vi "board_new_board.vi"() -> (0 "chess pieces":variant, 1 "new board":picture[][](array[picture]))   [LabVIEW 2014]
doc: "Generates an 8x8 array of pictures that depicts a chess board with pieces in their starting positions (white on bottom)."
uses:
  board_piece_names.ctl
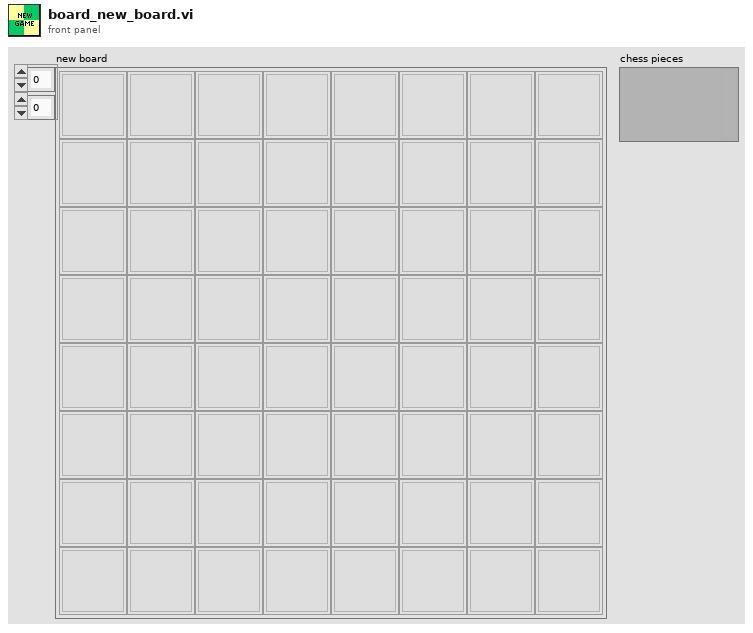
[diagram p1: front panel]
types:
  T1 = typedef "board_piece_names.ctl" = enum16{"Bblk", "Bwht", "Kblk", "Kwht", "Nblk", "Nwht", "Pblk", "Pwht", "Qblk", "Qwht", "Rblk", "Rwht"}
  T2 = typedef "imagedata.ctl" = cluster{"image type":i32, "image depth":i32, "image":u8[], "mask":u8[], "colors":u32[], "Rectangle":cluster{"left":i16, "top":i16, "right":i16, "bottom":i16}}
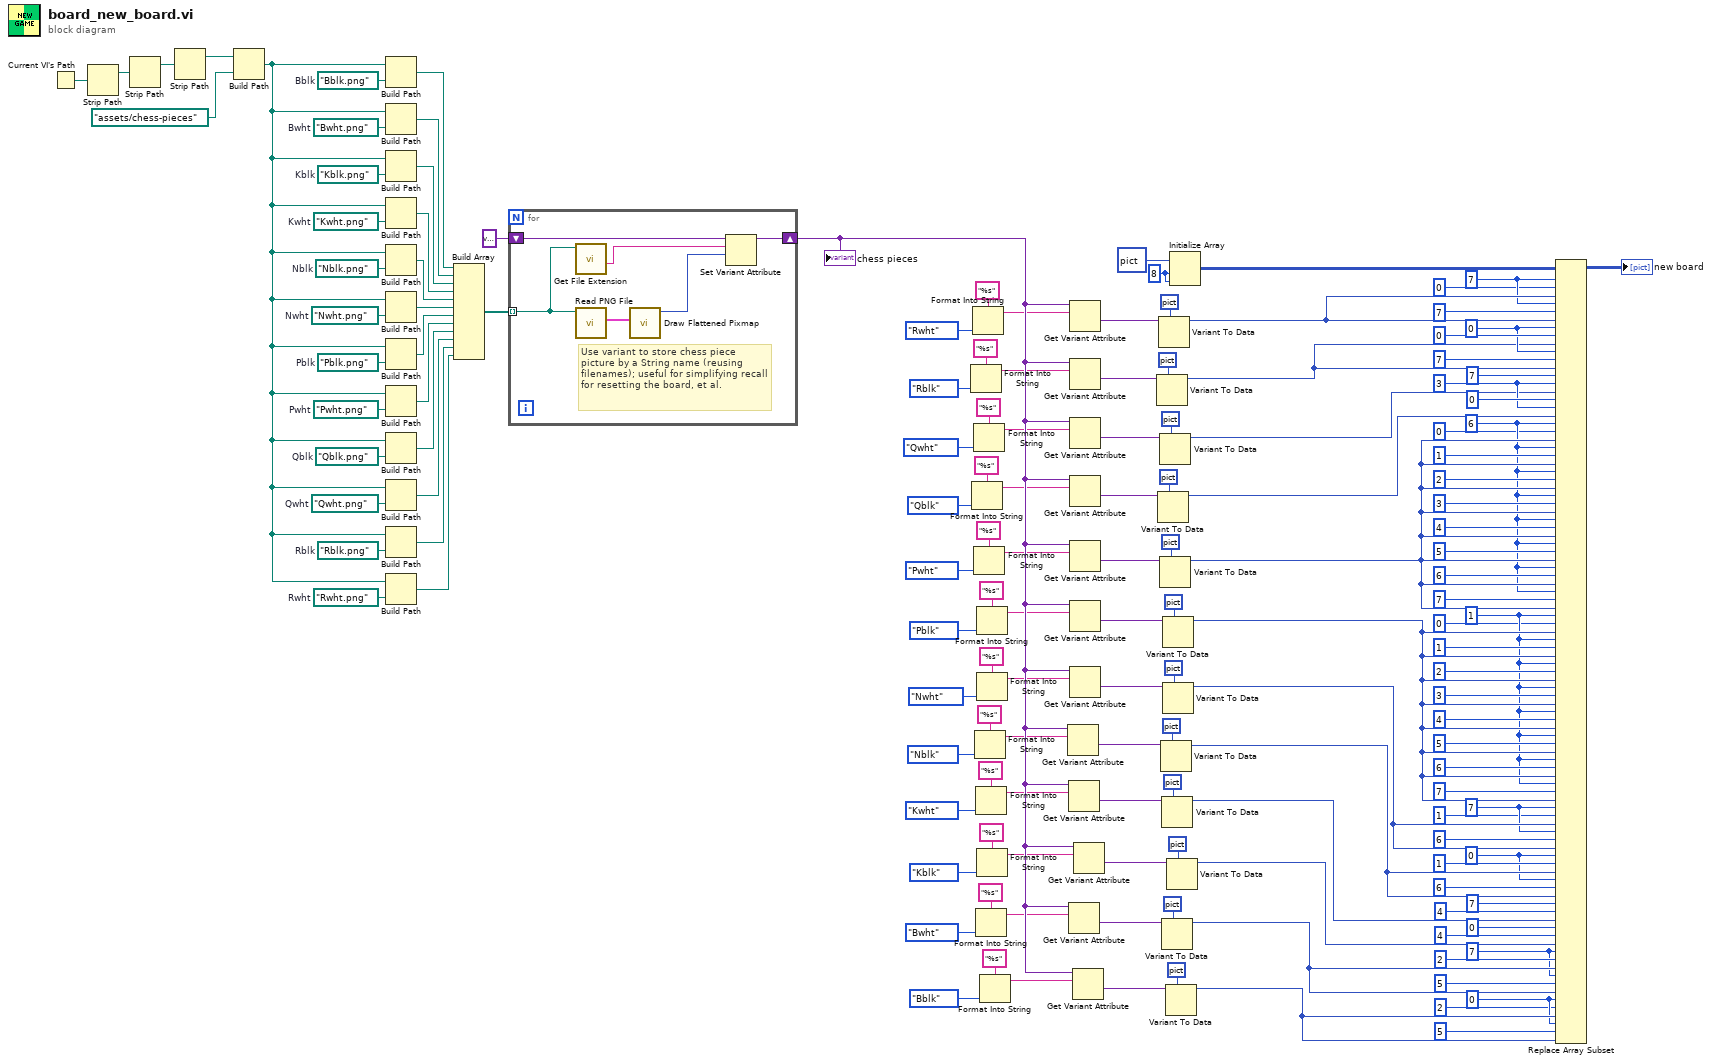
[diagram p0: block diagram]
diagram:
  w18 = path "Rwht.png"  # Rwht
  w19 = path "Rblk.png"  # Rblk
  w16 = path "Qwht.png"  # Qwht
  w20 = path "Qblk.png"  # Qblk
  w21 = path "Pwht.png"  # Pwht
  w15 = path "Pblk.png"  # Pblk
  w22 = path "Nwht.png"  # Nwht
  w23 = path "Nblk.png"  # Nblk
  w17 = path "Kwht.png"  # Kwht
  w24 = path "Kblk.png"  # Kblk
  w25 = path "Bwht.png"  # Bwht
  w28 = path "Bblk.png"  # Bblk
  w147 = 0
  w142 = 7
  w132 = 0
  w129 = 7
  w119 = 1 ("disabled index (col)")
  w109 = 6 ("disabled index (col)")
  w106 = 3 ("disabled index (col)")
  w100 = 0 ("index (row)")
  w40 = 8 ("dimension size")
  w42 = 7 ("index (row)")
  n1 = Current VI's Path() -> (path=w31:path)
  n2 = Strip Path(path=w31) -> (stripped path=w30:path)  [unwired: 1 out]
  n3 = Strip Path(path=w30) -> (stripped path=w27:path)  [unwired: 1 out]
  n4 = Strip Path(path=w27) -> (stripped path=w26:path)  [unwired: 1 out]
  n5 = Build Path(base path=w26, name or relative path=path "assets/chess-pieces") -> (appended path=w14:path)
  n6 = Build Path(base path=w14, name or relative path=w28) -> (appended path=w13:path)
  n7 = Build Path(base path=w14, name or relative path=w25) -> (appended path=w12:path)
  n8 = Build Path(base path=w14, name or relative path=w24) -> (appended path=w11:path)
  n9 = Build Path(base path=w14, name or relative path=w17) -> (appended path=w10:path)
  n10 = Build Path(base path=w14, name or relative path=w23) -> (appended path=w9:path)
  n11 = Build Path(base path=w14, name or relative path=w22) -> (appended path=w8:path)
  n12 = Build Path(base path=w14, name or relative path=w15) -> (appended path=w7:path)
  n13 = Build Path(base path=w14, name or relative path=w21) -> (appended path=w6:path)
  n14 = Build Path(base path=w14, name or relative path=w20) -> (appended path=w5:path)
  n15 = Build Path(base path=w14, name or relative path=w16) -> (appended path=w4:path)
  n16 = Build Path(base path=w14, name or relative path=w19) -> (appended path=w3:path)
  n17 = Build Path(base path=w14, name or relative path=w18) -> (appended path=w2:path)
  n18 = Build Array(w13, w12, w11, w10, w9, w8, w7, w6, w5, w4, w3, w2) -> (w1:path[])
  n19 = for {
    tunnel: w1 -> [w154] mode=indexing
    shift-right: [w156] -> w98
    shift-left: variant -> [w157]
    # "Use variant to store chess piece picture by a String name (reusing filenames); useful for simplifying recall for resetting the board, et al."
    n20 = call <vilib>:"Get File Extension.vi"("file"=w154) -> ("filename without extension"=w155:string)  [unwired: 6 in, 4 out]
    n21 = call <vilib>:"Read PNG File.vi"("path to PNG file"=w154) -> ("image data"=w158:T2)  [unwired: 8 in, 2 out]
    n22 = call <vilib>:"Draw Flattened Pixmap.vi"("image data"=w158) -> ("new picture"=w153:picture)  [unwired: 8 in]
    n23 = Set Variant Attribute(Variant=w157, name=w155, value=w153) -> (Variant out=w156:variant)  [unwired: 1 in, 2 out]
  }
  "chess pieces" <- w98
  n24 = Format Into String(format string="%s", board_piece_names."Rblk") -> (resulting string=w45:string)  [unwired: 2 in, 1 out]
  n25 = Format Into String(format string="%s", board_piece_names."Qblk") -> (resulting string=w55:string)  [unwired: 2 in, 1 out]
  n26 = Format Into String(format string="%s", board_piece_names."Rwht") -> (resulting string=w36:string)  [unwired: 2 in, 1 out]
  n27 = Format Into String(format string="%s", board_piece_names."Qwht") -> (resulting string=w50:string)  [unwired: 2 in, 1 out]
  n28 = Format Into String(format string="%s", board_piece_names."Pwht") -> (resulting string=w60:string)  [unwired: 2 in, 1 out]
  n29 = Format Into String(format string="%s", board_piece_names."Nblk") -> (resulting string=w75:string)  [unwired: 2 in, 1 out]
  n30 = Format Into String(format string="%s", board_piece_names."Kwht") -> (resulting string=w80:string)  [unwired: 2 in, 1 out]
  n31 = Format Into String(format string="%s", board_piece_names."Bwht") -> (resulting string=w90:string)  [unwired: 2 in, 1 out]
  n32 = Format Into String(format string="%s", board_piece_names."Pblk") -> (resulting string=w65:string)  [unwired: 2 in, 1 out]
  n33 = Format Into String(format string="%s", board_piece_names."Nwht") -> (resulting string=w70:string)  [unwired: 2 in, 1 out]
  n34 = Format Into String(format string="%s", board_piece_names."Kblk") -> (resulting string=w85:string)  [unwired: 2 in, 1 out]
  n35 = Format Into String(format string="%s", board_piece_names."Bblk") -> (resulting string=w95:string)  [unwired: 2 in, 1 out]
  n36 = Get Variant Attribute(Variant=w98, name=w75) -> (value=w74:variant)  [unwired: 2 in, 3 out]
  n37 = Get Variant Attribute(Variant=w98, name=w80) -> (value=w81:variant)  [unwired: 2 in, 3 out]
  n38 = Get Variant Attribute(Variant=w98, name=w90) -> (value=w91:variant)  [unwired: 2 in, 3 out]
  n39 = Get Variant Attribute(Variant=w98, name=w36) -> (value=w37:variant)  [unwired: 2 in, 3 out]
  n40 = Get Variant Attribute(Variant=w98, name=w45) -> (value=w44:variant)  [unwired: 2 in, 3 out]
  n41 = Get Variant Attribute(Variant=w98, name=w50) -> (value=w51:variant)  [unwired: 2 in, 3 out]
  n42 = Get Variant Attribute(Variant=w98, name=w55) -> (value=w54:variant)  [unwired: 2 in, 3 out]
  n43 = Get Variant Attribute(Variant=w98, name=w60) -> (value=w61:variant)  [unwired: 2 in, 3 out]
  n44 = Get Variant Attribute(Variant=w98, name=w65) -> (value=w64:variant)  [unwired: 2 in, 3 out]
  n45 = Get Variant Attribute(Variant=w98, name=w70) -> (value=w71:variant)  [unwired: 2 in, 3 out]
  n46 = Get Variant Attribute(Variant=w98, name=w95) -> (value=w94:variant)  [unwired: 2 in, 3 out]
  n47 = Get Variant Attribute(Variant=w98, name=w85) -> (value=w84:variant)  [unwired: 2 in, 3 out]
  n48 = Variant To Data(type=picture data[5B] ("new picture"), Variant=w44) -> (data=w99:picture)  [unwired: 1 in, 1 out]
  n49 = Variant To Data(type=picture data[5B] ("new picture"), Variant=w54) -> (data=w104:picture)  [unwired: 1 in, 1 out]
  n50 = Variant To Data(type=picture data[5B] ("new picture"), Variant=w37) -> (data=w152:picture)  [unwired: 1 in, 1 out]
  n51 = Variant To Data(type=picture data[5B] ("new picture"), Variant=w51) -> (data=w105:picture)  [unwired: 1 in, 1 out]
  n52 = Variant To Data(type=picture data[5B] ("new picture"), Variant=w61) -> (data=w117:picture)  [unwired: 1 in, 1 out]
  n53 = Variant To Data(type=picture data[5B] ("new picture"), Variant=w74) -> (data=w135:picture)  [unwired: 1 in, 1 out]
  n54 = Variant To Data(type=picture data[5B] ("new picture"), Variant=w81) -> (data=w140:picture)  [unwired: 1 in, 1 out]
  n55 = Variant To Data(type=picture data[5B] ("new picture"), Variant=w91) -> (data=w145:picture)  [unwired: 1 in, 1 out]
  n56 = Variant To Data(type=picture data[5B] ("new picture"), Variant=w64) -> (data=w127:picture)  [unwired: 1 in, 1 out]
  n57 = Variant To Data(type=picture data[5B] ("new picture"), Variant=w71) -> (data=w131:picture)  [unwired: 1 in, 1 out]
  n58 = Variant To Data(type=picture data[5B] ("new picture"), Variant=w94) -> (data=w149:picture)  [unwired: 1 in, 1 out]
  n59 = Variant To Data(type=picture data[5B] ("new picture"), Variant=w84) -> (data=w141:picture)  [unwired: 1 in, 1 out]
  n60 = Initialize Array(picture data[5B] ("65x65 blank"), w40, w40) -> (w41:picture[][])
  n61 = Replace Array Subset(array=w41, new element #1=w152, index (row) #1=w42, index (col) #1=0 ("disabled index (col)"), new element #2=w152, index (row) #2=w42, index (col) #2=7 ("index (row)"), new element #3=w99, index (row) #3=w100, index (col) #3=0 ("index (row)"), new element #4=w99, index (row) #4=w100, index (col) #4=7 ("index (row)"), new element #5=w105, index (row) #5=7 ("index (row)"), index (col) #5=w106, new element #6=w104, index (row) #6=0 ("disabled index (col)"), index (col) #6=w106, new element #7=w117, index (row) #7=w109, index (col) #7=0 ("disabled index (col)"), new element #8=w117, index (row) #8=w109, index (col) #8=1 ("disabled index (col)"), new element #9=w117, index (row) #9=w109, index (col) #9=2 ("disabled index (col)"), new element #10=w117, index (row) #10=w109, index (col) #10=3 ("disabled index (col)"), new element #11=w117, index (row) #11=w109, index (col) #11=4 ("disabled index (col)"), new element #12=w117, index (row) #12=w109, index (col) #12=5 ("disabled index (col)"), new element #13=w117, index (row) #13=w109, index (col) #13=6 ("disabled index (col)"), new element #14=w117, index (row) #14=w109, index (col) #14=7 ("disabled index (col)"), new element #15=w127, index (row) #15=w119, index (col) #15=0 ("disabled index (col)"), new element #16=w127, index (row) #16=w119, index (col) #16=1 ("disabled index (col)"), new element #17=w127, index (row) #17=w119, index (col) #17=2 ("disabled index (col)"), new element #18=w127, index (row) #18=w119, index (col) #18=3 ("disabled index (col)"), new element #19=w127, index (row) #19=w119, index (col) #19=4 ("disabled index (col)"), new element #20=w127, index (row) #20=w119, index (col) #20=5 ("disabled index (col)"), new element #21=w127, index (row) #21=w119, index (col) #21=6 ("disabled index (col)"), new element #22=w127, index (row) #22=w119, index (col) #22=7 ("disabled index (col)"), new element #23=w131, index (row) #23=w129, index (col) #23=1, new element #24=w131, index (row) #24=w129, index (col) #24=6, new element #25=w135, index (row) #25=w132, index (col) #25=1, new element #26=w135, index (row) #26=w132, index (col) #26=6, new element #27=w140, index (row) #27=7, index (col) #27=4, new element #28=w141, index (row) #28=0, index (col) #28=4, new element #29=w145, index (row) #29=w142, index (col) #29=2, new element #30=w145, index (row) #30=w142, index (col) #30=5, new element #31=w149, index (row) #31=w147, index (col) #31=2, new element #32=w149, index (row) #32=w147, index (col) #32=5) -> (→"new board":picture[][])
